vi "shutter vi_coMD.vi"() -> ()   [LabVIEW 2012]
doc: "SciScan 1.2 160622"
uses:
  <vilib>/DAQmx/write.llb/DAQmx Write (Digital Bool 1Line 1Point).vi
  GFG/GFGstringGet.vi
  <vilib>/DAQmx/create/channels.llb/DAQmx Create Channel (DO-Digital Output).vi
  GFG/GFGbooleanGet.vi
  <vilib>/DAQmx/miscellaneous.llb/DAQmx Fill In Error Info.vi
  GFG/GFGfpRefGet.vi
  GFG/GFG library.lvlib
panel:
  out "error out":errorcluster
  in  "Clear":bool
  out "Source VI":string
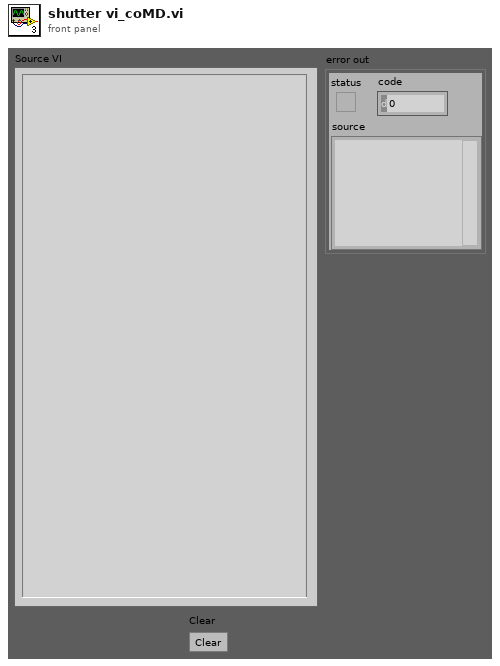
[diagram p1: front panel]
types:
  T1 = enum8{"Enabled", "Disabled", "Disabled and Grayed Out"}
  T2 = cluster{"WaveformChartRef":refnum<vi>, "DigitalRef":refnum<vi>, "ArrayRef":refnum<vi>, "TabControlRef":refnum<vi>, "EnumRef":refnum<vi>, "RingRef":refnum<vi>, "BooleanRef":refnum<vi>, "KnobRef":refnum<vi>, "SlideRef":refnum<vi>, "PathRef":refnum<vi>, "StringRef":refnum<vi>, "ComboBox":refnum<vi>, "WaveformGraphRef":refnum<vi>}
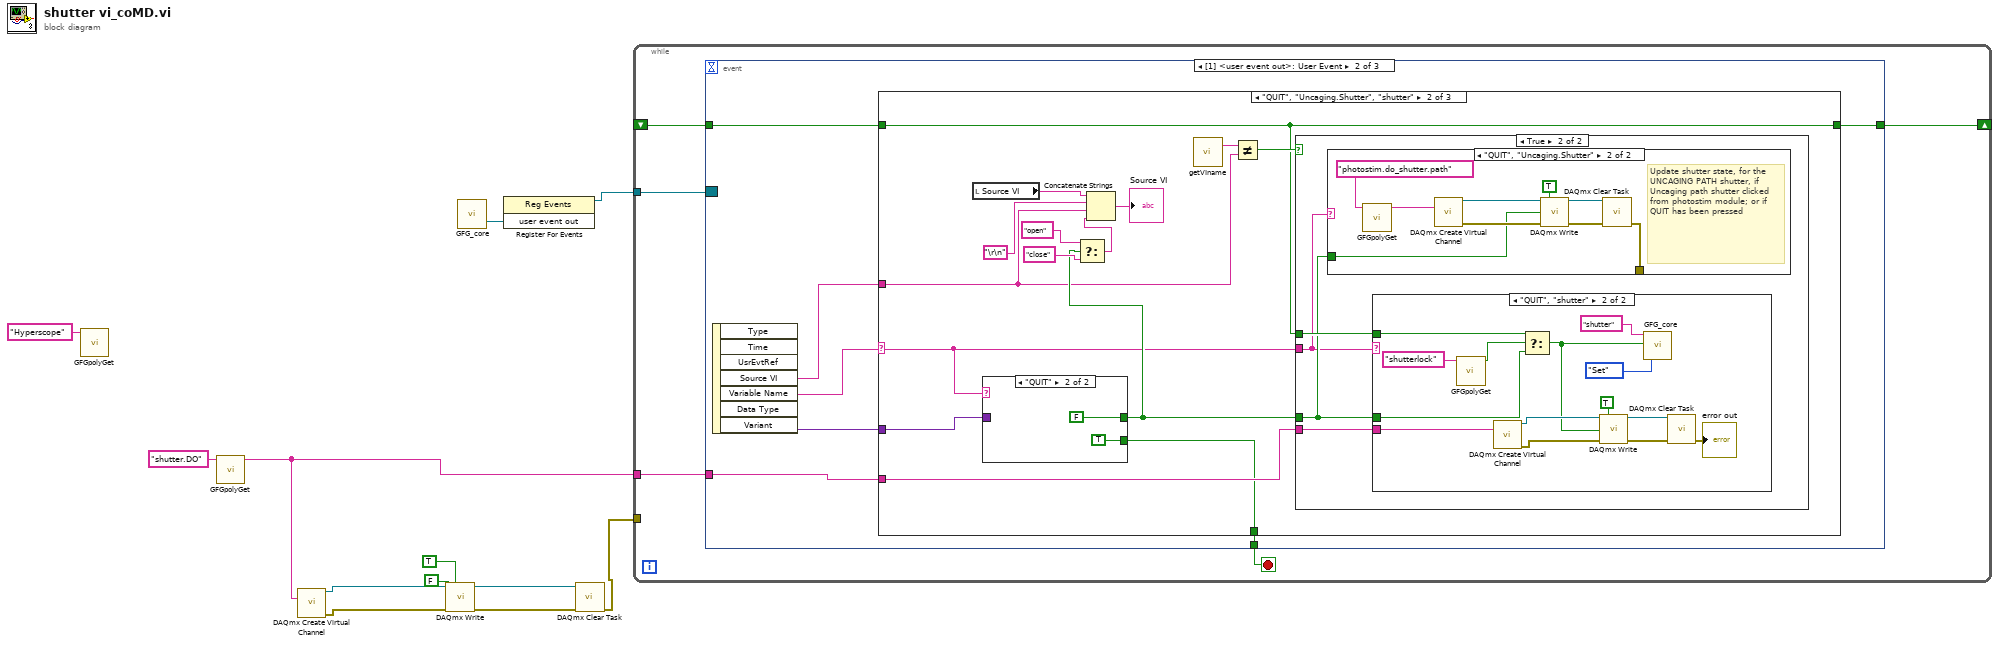
[diagram p0: block diagram]
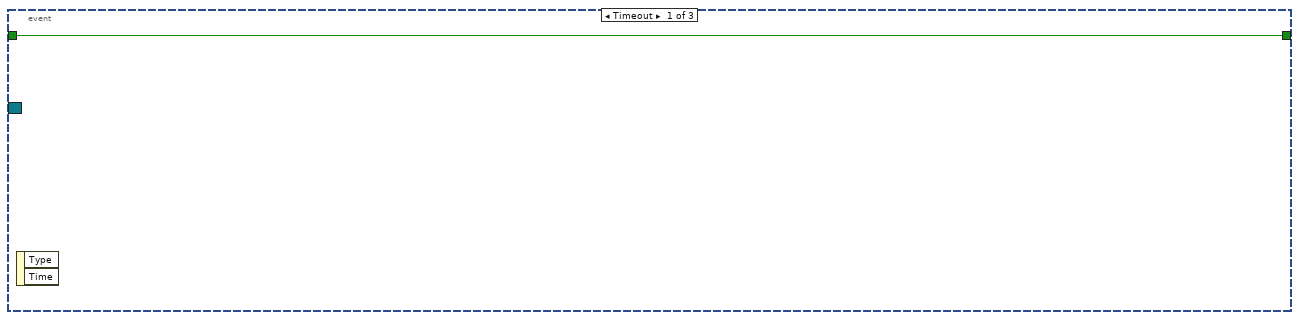
[diagram p2: hidden frame]
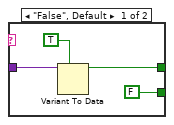
[diagram p7: hidden frame]
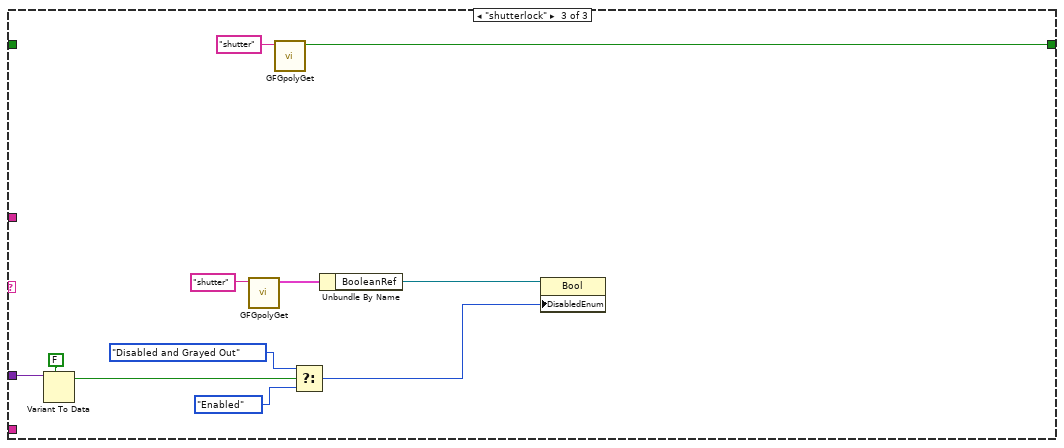
[diagram p8: hidden frame]
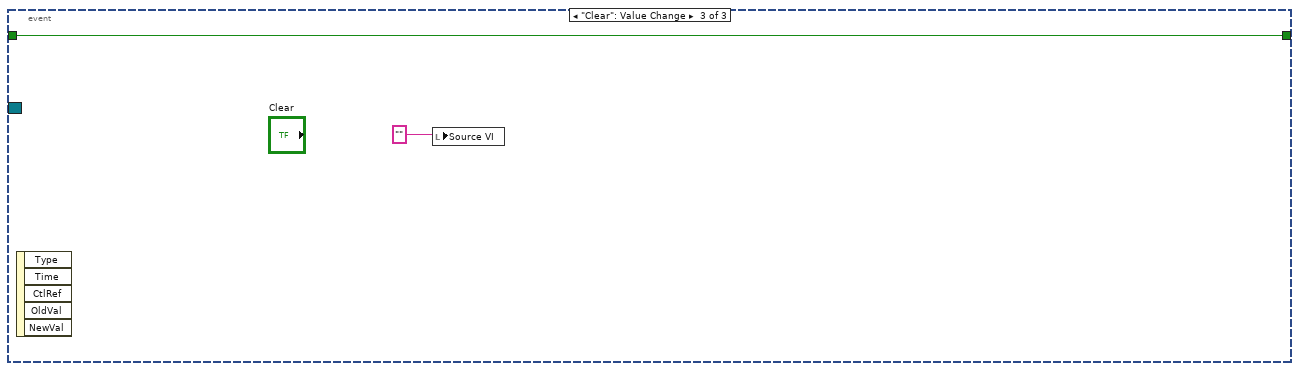
[diagram p9: hidden frame]
diagram:
  n1 = call-poly "GFGpolyGet.vi"("Variable Name in"="Hyperscope" ("Tag in")) -> ()  [unwired: 9 in, 2 out]
  n2 = call-poly "GFGpolyGet.vi"("Variable Name in"="shutter.DO" ("Tag in")) -> ("String"=w4:string)  [unwired: 9 in, 1 out]
  n3 = call-poly <vilib>:"DAQmx Create Virtual Channel.vi"("lines"=w4) -> ("task out"=w5:refnum<k21>, "error out"=w9:errorcluster)  [unwired: 13 in]
  n4 = call-poly <vilib>:"DAQmx Write.vi"("task/channels in"=w5, "auto start"=TRUE, "data"=FALSE, "error in"=w9) -> ("task out"=w7:refnum<k21>, "error out"=w8:errorcluster)  [unwired: 9 in, 1 out]
  n5 = call "GFG_core.vi"() -> ("user event out"=w12:refnum<user-event>)  [unwired: 13 in, 6 out]
  n6 = register-events(w12) -> (reference out=w11:refnum<event-registration>)  [unwired: 2 in, 1 out]
  n7 = call <vilib>:"DAQmx Clear Task.vi"("task in"=w7, "error in"=w8) -> ("error out"=w2:errorcluster)  [unwired: 13 in]
  n8 = while {
    tunnel: w11 -> [w17]
    tunnel: w4 -> [w15]
    tunnel: w2 -> [_]
    shift-right: [w14] -> _
    shift-left: _ -> [w13]
    stop <- w16 stop-if-true
    n9 = event shown="[1] <user event out>: User Event" {
      selector: w17 -> [_ _ _]
      dyn-events: _ -> [_ _ _]
      timeout: _ -> [_ _ _]
      tunnel: [_ w22 _] -> w16
      tunnel: w15 -> [_ w23 _]
      tunnel: [w18 w20 w86] -> w14
      tunnel: w13 -> [w18 w19 w86]
      event Timeout {
        n10 = event-data() -> ()  [unwired: 1 in, 2 out]
      }
      event User Event {
        n11 = event-data() -> ("Source VI"=w21:string, "Variable Name"=w25:string, "Variant"=w24:variant)  [unwired: 1 in, 4 out]
        n12 = case shown="\"QUIT\", \"Uncaging.Shutter\", \"shutter\"" w25 {
          selector: w25 -> [_ w27 _]
          tunnel: w24 -> [_ w41 w75]
          tunnel: w23 -> [_ w40 _]
          tunnel: [_ w39 _] -> w22
          tunnel: w21 -> [_ w30 _]
          tunnel: [w26 w28 w76] -> w20
          tunnel: w19 -> [w26 w28 _]
          frame "False", Default {
          }
          frame "QUIT", "Uncaging.Shutter", "shutter" {
            n13 = local read "Source VI"() -> (w38:string)
            n14 = case shown="\"QUIT\"" w27 {
              tunnel: w41 -> [w72 _]
              tunnel: [w70 FALSE] -> w33
              tunnel: [FALSE TRUE] -> w39
              frame "False", Default {
                n15 = Variant To Data(type=TRUE, Variant=w72) -> (data=w70:bool)  [unwired: 1 in, 1 out]
              }
              frame "QUIT" {
              }
            }
            n16 = Select(t="open" ("Source VI"), s=w33, f="close" ("Source VI")) -> (s? t:f=w32:string)
            n17 = Concatenate Strings(w38, "\r\n", w30, w32) -> (→"Source VI":string)
            n18 = call "getVIname.vi"() -> ("VI name"=w31:string)  [unwired: 19 in]
            n19 = Not Equal?(x=w31, y=w30) -> (x != y?=w29:bool)
            n20 = case shown="True" w29 {
              tunnel: w40 -> [_ w45]
              tunnel: w33 -> [_ w43]
              tunnel: w28 -> [_ w44]
              tunnel: w27 -> [_ w42]
              frame False {
              }
              frame True {
                n21 = case shown="\"QUIT\", \"Uncaging.Shutter\"" w42 {
                  tunnel: w43 -> [_ w63]
                  tunnel: [_ w65] -> _
                  frame "False", Default {
                  }
                  frame "QUIT", "Uncaging.Shutter" {
                    # "Update shutter state, for the UNCAGING PATH shutter, if Uncaging path shutter clicked from photostim module; or if QUIT has been pressed"
                    n22 = call-poly "GFGpolyGet.vi"("Variable Name in"="photostim.do_shutter.path") -> ("String"=w64:string)  [unwired: 9 in, 1 out]
                    n23 = call-poly <vilib>:"DAQmx Create Virtual Channel.vi"("lines"=w64) -> ("task out"=w62:refnum<k21>, "error out"=w67:errorcluster)  [unwired: 13 in]
                    n24 = call-poly <vilib>:"DAQmx Write.vi"("task/channels in"=w62, "auto start"=TRUE, "data"=w63, "error in"=w67) -> ("task out"=w61:refnum<k21>, "error out"=w66:errorcluster)  [unwired: 9 in, 1 out]
                    n25 = call <vilib>:"DAQmx Clear Task.vi"("task in"=w61, "error in"=w66) -> ("error out"=w65:errorcluster)  [unwired: 13 in]
                  }
                }
                n26 = case shown="\"QUIT\", \"shutter\"" w42 {
                  tunnel: w45 -> [_ w59]
                  tunnel: w44 -> [_ w50]
                  tunnel: w43 -> [_ w46]
                  frame "False", Default {
                  }
                  frame "QUIT", "shutter" {
                    n27 = call-poly "GFGpolyGet.vi"("Variable Name in"="shutterlock") -> ("Boolean Value OUT"=w51:bool)  [unwired: 9 in, 1 out]
                    n28 = call-poly <vilib>:"DAQmx Create Virtual Channel.vi"("lines"=w59) -> ("task out"=w58:refnum<k21>, "error out"=w54:errorcluster)  [unwired: 13 in]
                    n29 = Select(t=w50, s=w51, f=w46) -> (s? t:f=w47:bool)
                    n30 = call-poly <vilib>:"DAQmx Write.vi"("task/channels in"=w58, "auto start"=TRUE, "data"=w47, "error in"=w54) -> ("task out"=w56:refnum<k21>, "error out"=w55:errorcluster)  [unwired: 9 in, 1 out]
                    n31 = call "GFG_core.vi"("Variable Name in"="shutter", "Variant in"=w47, "Action"=enum16{"Init", "Set", "Get", "Clear"}."Set") -> ()  [unwired: 10 in, 7 out]
                    n32 = call <vilib>:"DAQmx Clear Task.vi"("task in"=w56, "error in"=w55) -> ("error out"=→"error out":errorcluster)  [unwired: 13 in]
                  }
                }
              }
            }
          }
          frame "shutterlock" {
            n33 = Variant To Data(type=FALSE, Variant=w75) -> (data=w83:bool)  [unwired: 1 in, 1 out]
            n34 = call-poly "GFGpolyGet.vi"("Variable Name in"="shutter") -> ("output cluster"=w77:T2)  [unwired: 9 in, 1 out]
            n35 = call-poly "GFGpolyGet.vi"("Variable Name in"="shutter") -> ("Boolean Value OUT"=w76:bool)  [unwired: 9 in, 1 out]
            n36 = Select(t=T1."Disabled and Grayed Out" ("Disabled"), s=w83, f=T1."Enabled" ("Disabled")) -> (s? t:f=w80:T1)
            n37 = Unbundle By Name(w77) -> ("BooleanRef"=w85:refnum<vi>)
            n38 = property class="Bool"(reference=w85, "DisabledEnum"=w80) -> ()  [unwired: 1 in, 2 out]
          }
        }
      }
      event "Clear": Value Change {
        n39 = event-data() -> ()  [unwired: 1 in, 5 out]
        n40 = local write "Source VI"("" ("Source VI")) -> ()
      }
    }
  }
